vi "Gen_RS_slot1_2.vi"(0 "appended path":path, 1 "prb_num":dbl, 2 "UL_subframe_num":dbl, 3 "cellid":dbl, 4 "error in (no error)":errorcluster caption="错误输入（无错误）") -> (5 "rs_slot1":cdb[](array[numeric]), 6 "rs_slot2":cdb[](array[numeric]), 7 "error IO":errorcluster)   [LabVIEW 2015]
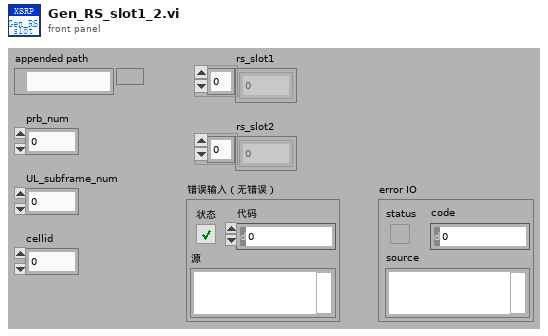
[diagram p1: front panel]
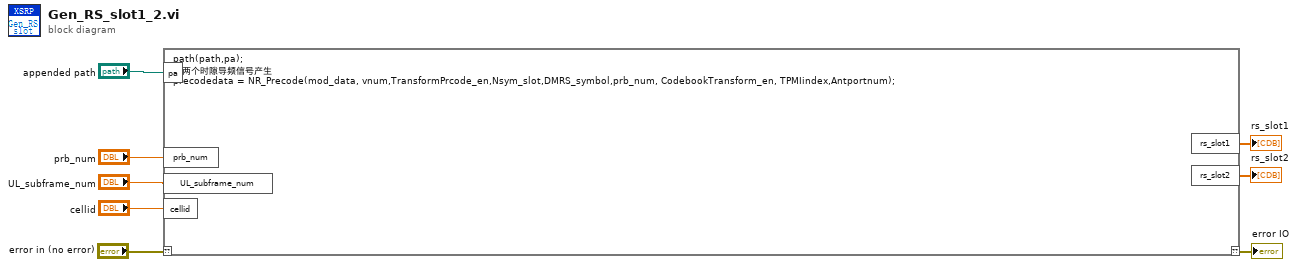
[diagram p0: block diagram]
diagram:
  n1 = script code="path(path,pa);\n%两个时隙导频信号产生\nprecodedata = NR_Precode(mod_data, vnum,TransformPrcode_en,Nsym_slot,DMRS_symbol,prb_num, CodebookTransform_en, TPMIindex,Antportnum);"("??"="error in (no error)", "pa"="appended path", "prb_num"="prb_num", "UL_subframe_num"="UL_subframe_num", "cellid"="cellid") -> ("??"=→"error IO":errorcluster, "rs_slot1"=→"rs_slot1":cdb[], "rs_slot2"=→"rs_slot2":cdb[])
